vi "AlazarCoprocessorRegisterRead.vi"(0 "Handle":u64, 1 "Offset":u32, 2 "error in (no error)":errorcluster) -> (3 "Handle":u64, 4 "Value":u32, 5 "Return Code":u32, 6 "error out":errorcluster)   [LabVIEW 2018]
doc: "Read the contents of a user-programmable coprocessor FPGA register."
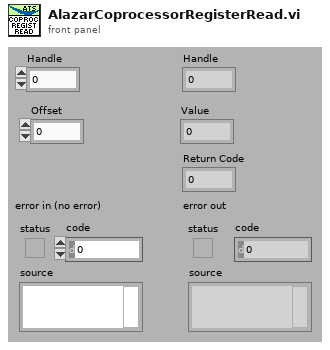
[diagram p1: front panel]
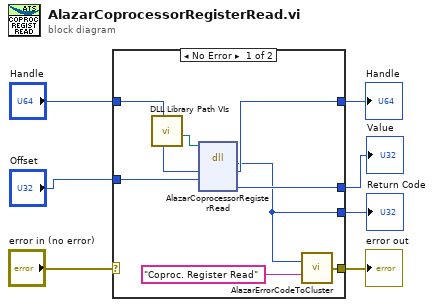
[diagram p0: block diagram]
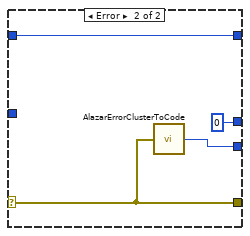
[diagram p2: hidden frame]
diagram:
  n1 = case shown="No Error" "error in (no error)" {
    selector: "error in (no error)" -> [_ w19]
    tunnel: [w11 w19] -> w6
    tunnel: [w10 w18] -> w5
    tunnel: "Handle" -> [w15 w17]
    tunnel: [w14 w17] -> w3
    tunnel: [w13 u32 0] -> w2
    tunnel: "Offset" -> [w12 _]
    frame No Error {
      n2 = call "DLL Library Path VIs.vi"() -> ("Alazar"=w8:path)  [unwired: 9 in, 2 out]
      n3 = dll-call lib="C:/Project/SerialSectOCT - FFT GPU/SerialSectOCT/Labview Software/DLL/ATSApi.dll" fn="AlazarCoprocessorRegisterRead"(path in=w8, "handle"=w15, "offset"=w12) -> ("return type"=w10:u32, "handle"=w14:u64, "value"=w13:u32)  [unwired: 4 in, 2 out]
      n4 = call "AlazarErrorCodeToCluster.vi"("Message"="Coproc. Register Read", "Error Code"=w10) -> ("error out"=w11:errorcluster)
    }
    frame Error {
      n5 = call "AlazarErrorClusterToCode.vi"("error in (no error)"=w19) -> ("Error Code"=w18:u32)
    }
  }
  "Handle" <- w3
  "error out" <- w6
  "Return Code" <- w5
  "Value" <- w2
